vi "Display Result.vi"() -> ()   [LabVIEW 2018]
panel:
  in  "frequency list Input":T1(array[cluster])=[{"frequency [Hz]"=200.0, "amplitude [V]"=0.5}, {"frequency [Hz]"=224.0, "amplitude [V]"=0.9}, {"frequency [Hz]"=250.0, "amplitude [V]"=2.5}, {"frequency [Hz]"=280.0, "amplitude [V]"=2.7}, {"frequency [Hz]"=315.0, "amplitude [V]"=2.0}, {"frequency [Hz]"=355.0, "amplitude [V]"=2.0}, {"frequency [Hz]"=400.0, "amplitude [V]"=3.8}, {"frequency [Hz]"=450.0, "amplitude [V]"=6.9}, {"frequency [Hz]"=500.0, "amplitude [V]"=9.7}, {"frequency [Hz]"=560.0, "amplitude [V]"=6.4}, {"frequency [Hz]"=630.0, "amplitude [V]"=6.5}, {"frequency [Hz]"=710.0, "amplitude [V]"=7.0}, {"frequency [Hz]"=800.0, "amplitude [V]"=7.0}, {"frequency [Hz]"=900.0, "amplitude [V]"=2.0}, {"frequency [Hz]"=1000.0, "amplitude [V]"=2.0}, {"frequency [Hz]"=1120.0, "amplitude [V]"=2.0}, {"frequency [Hz]"=1250.0, "amplitude [V]"=2.0}, {"frequency [Hz]"=1400.0, "amplitude [V]"=2.0}, {"frequency [Hz]"=1600.0, "amplitude [V]"=4.0}, {"frequency [Hz]"=1800.0, "amplitude [V]"=1.5}, {"frequency [Hz]"=2000.0, "amplitude [V]"=1.2}, {"frequency [Hz]"=2240.0, "amplitude [V]"=1.2}, {"frequency [Hz]"=2500.0, "amplitude [V]"=1.1}, {"frequency [Hz]"=2800.0, "amplitude [V]"=1.0}, {"frequency [Hz]"=3150.0, "amplitude [V]"=1.0}, {"frequency [Hz]"=3550.0, "amplitude [V]"=1.8}, {"frequency [Hz]"=4000.0, "amplitude [V]"=2.2}, {"frequency [Hz]"=4500.0, "amplitude [V]"=6.0}, {"frequency [Hz]"=5000.0, "amplitude [V]"=1.8}, {"frequency [Hz]"=5600.0, "amplitude [V]"=3.2}, {"frequency [Hz]"=6300.0, "amplitude [V]"=2.2}, {"frequency [Hz]"=7100.0, "amplitude [V]"=8.0}, {"frequency [Hz]"=8000.0, "amplitude [V]"=1.1}]
  in  "Response Level 2":cluster{"frequency":dbl[], "magnitude":dbl[]}(graph) caption="Mic 1Response Level"
  in  "Response Level 1":cluster{"frequency":dbl[], "magnitude":dbl[]}(graph) caption="Mic 1Response Level"
  out "Table":string[][](table)
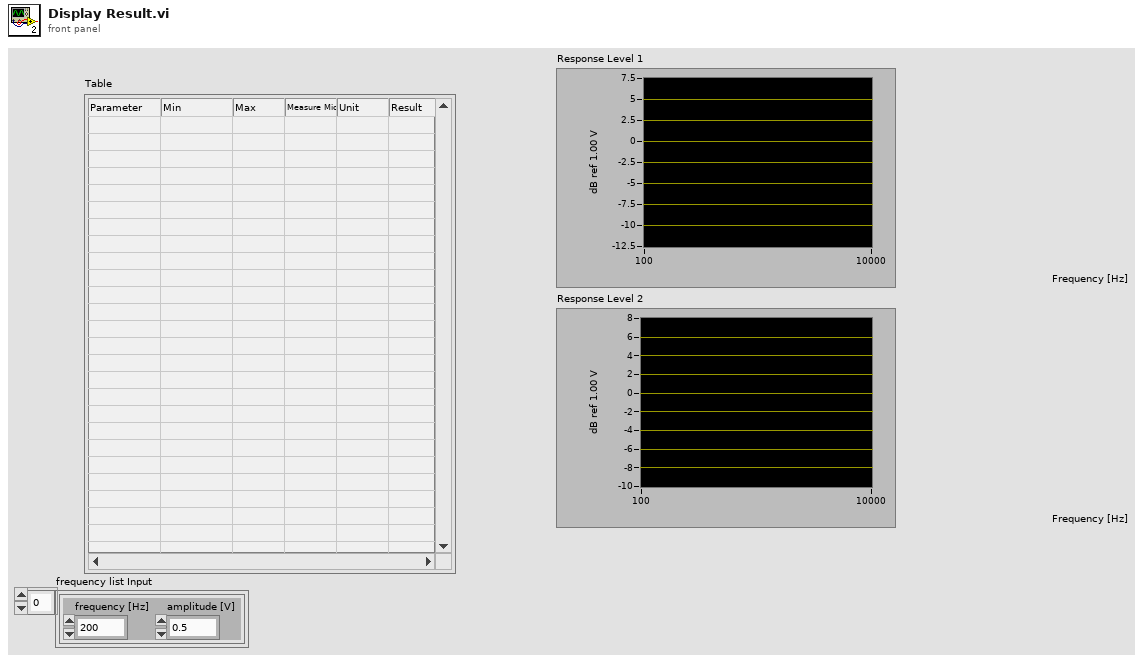
[diagram p1: front panel]
types:
  T1 = cluster{"frequency [Hz]":dbl, "amplitude [V]":dbl}[]
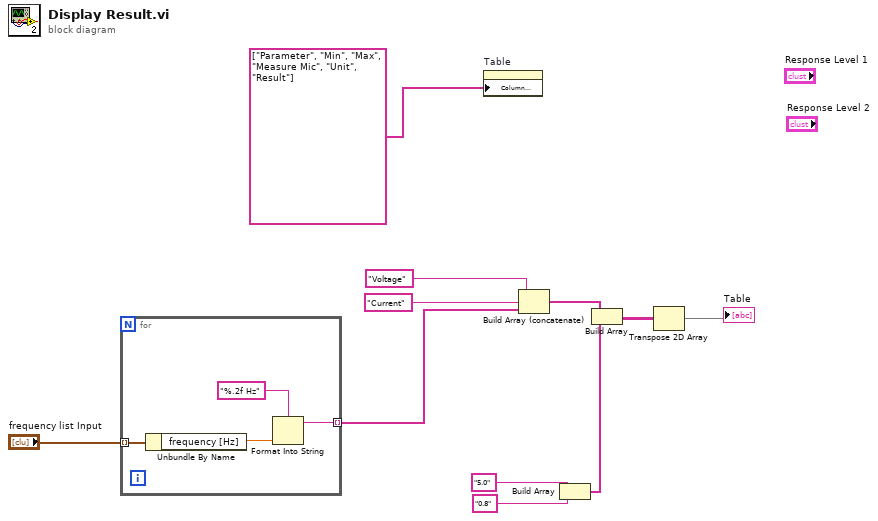
[diagram p0: block diagram]
diagram:
  n1 = for {
    tunnel: "frequency list Input" -> [w15] mode=indexing
    tunnel: [w12] -> w1 mode=indexing
    n2 = Unbundle By Name(w15) -> ("frequency [Hz]"=w13:dbl)
    n3 = Format Into String(format string="%.2f Hz", w13) -> (resulting string=w12:string)  [unwired: 2 in, 1 out]
  }
  n4 = property on="Table" class="Tbl (strict)"("Column Headers[]"=string[] ["Parameter", "Min", "Max", "Measure Mic", "Unit", "Result"] ("Column Header Strings[]")) -> ()  [unwired: 2 in, 2 out]
  n5 = Build Array (concatenate)("Voltage", "Current", w1) -> (w7:string[])
  n6 = Build Array("5.0", "0.8") -> (w6:string[])
  n7 = Build Array(w7, w6) -> (w5:string[][])
  n8 = Transpose 2D Array(2D array=w5) -> (transposed array=→"Table":string[][])
